vi "Encoded 2D gaussian.vi"(5 "Coefficients":dbl[](array[numeric]) format="%.5f", 6 "X":dbl format="%.3f", 7 "code":dbl format="%.2f", 8 "fit type":u16, 9 "Flag":enum16{"no deriv", "deriv"}(ring)) -> (0 "Derivatives":dbl[](array[numeric]) format="%.5f", 2 "Y":dbl format="%.3f")   [LabVIEW 2011]
doc: "Evaluates the fit function at a point given the specified coefficients (i.e., fit parameters). Code is the value used to convert a raster-encoded 2-D position (which is what is supplied to this function by its caller) into a true 2-D position (which is what the equations for the function need to use).\n\nIf the partial derivatives of the function are known, the user also furnishes the equations for the partial derivatives of this function with respect to each coefficient. The input control Flag should then be set to 1 (deriv) by all calling VIs.\n\nIf the partial derivatives of the function are not known, the input control Flag should be set to 0 (no deriv) by all calling VIs, and a numerical approximation to the partial derivatives will be computed."
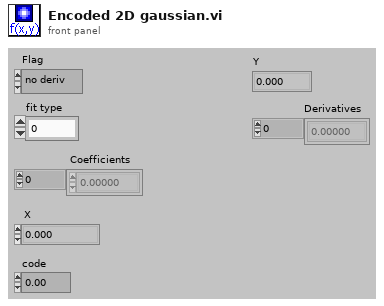
[diagram p1: front panel]
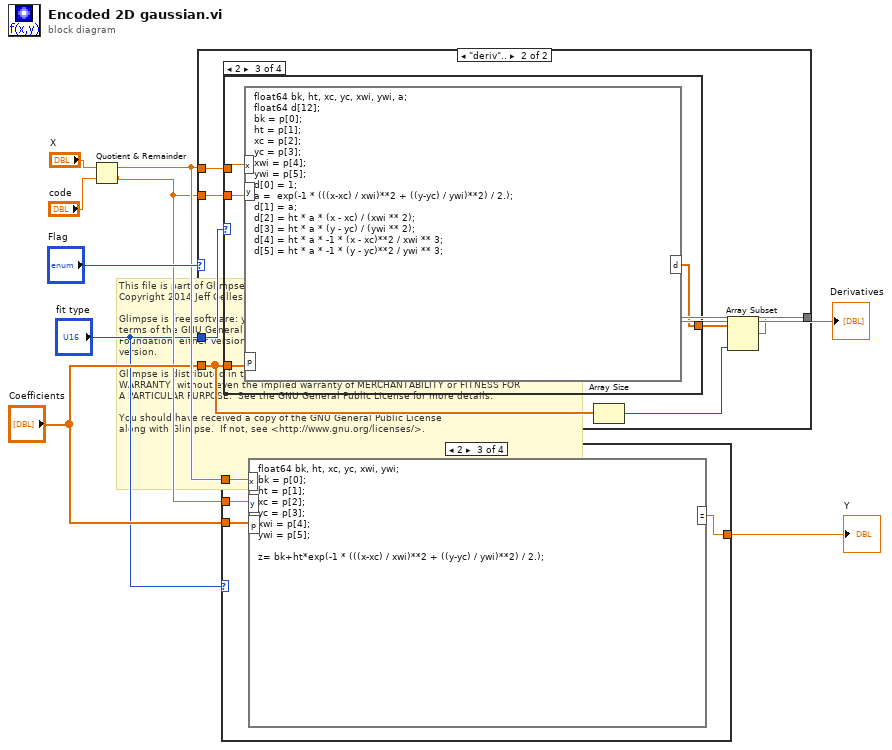
[diagram p0: block diagram]
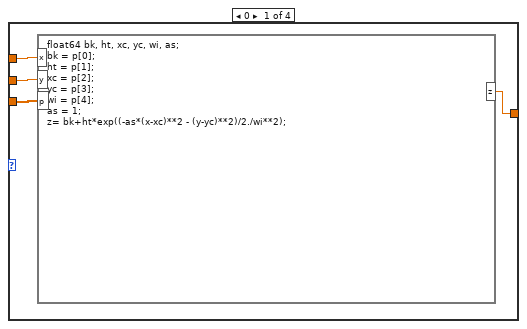
[diagram p2: hidden frame]
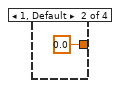
[diagram p3: hidden frame]
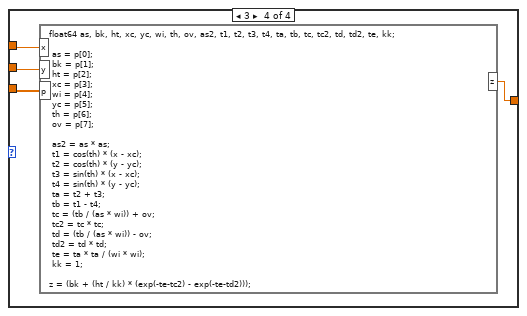
[diagram p4: hidden frame]
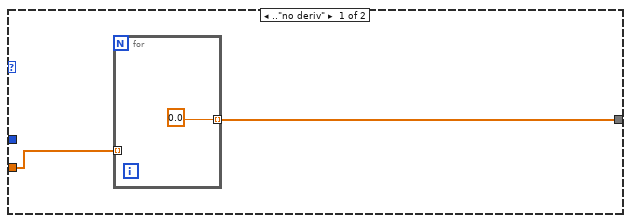
[diagram p5: hidden frame]
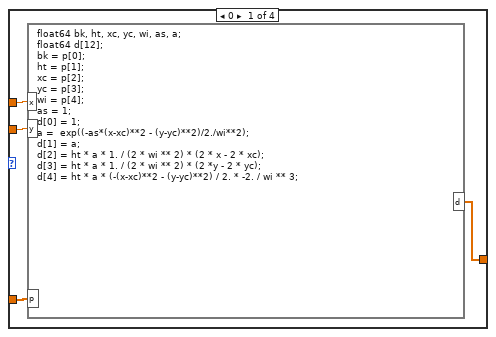
[diagram p6: hidden frame]
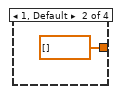
[diagram p7: hidden frame]
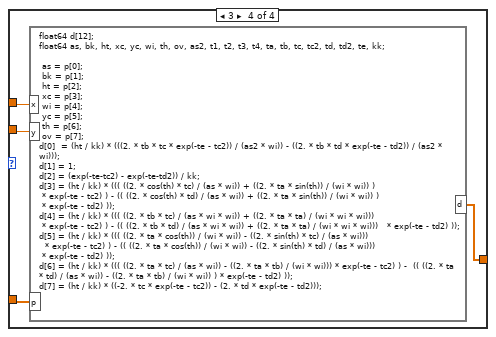
[diagram p8: hidden frame]
diagram:
  # "This file is part of Glimpse. \nCopyright 2014 Jeff Gelles, Brandeis University.    \n\nGlimpse is free software: you can redistribute it and/or modify it under the \nterms of the GNU General Public License as published by the Free Software \nFoundation, either version 3 of the License, or (at your option) any later \nversion.\n\nGlimpse is distributed in the hope that it will be useful, but WITHOUT ANY \nWARRANTY; without even the implied warranty of MERCHANTABILITY or FITNESS FOR \nA PARTICULAR PURPOSE.  See the GNU General Public License for more details.\n\nYou should have received a copy of the GNU General Public License\nalong with Glimpse.  If not, see <http://www.gnu.org/licenses/>."
  n1 = Quotient & Remainder(x="X", y="code") -> (x-y*floor(x/y)=w5:dbl, floor(x/y)=w2:dbl)
  n2 = case shown="\"deriv\".." "Flag" {
    tunnel: w5 -> [_ w19]
    tunnel: "Coefficients" -> [w11 w17]
    tunnel: [w10 w14] -> w3
    tunnel: w2 -> [_ w18]
    tunnel: "fit type" -> [_ w13]
    frame .."no deriv" {
      n3 = for {
        tunnel: w11 -> [_] mode=indexing
        tunnel: [0.0] -> w10 mode=indexing
      }
    }
    frame "deriv".. {
      n4 = case shown="2" w13 {
        tunnel: w19 -> [w23 _ w28 w32]
        tunnel: w18 -> [w22 _ w27 w31]
        tunnel: w17 -> [w21 _ w26 w30]
        tunnel: [w20 dbl[] [] w25 w29] -> w15
        frame 0 {
          n5 = formula code="float64 bk, ht, xc, yc, wi, as, a;\nfloat64 d[12];\nbk = p[0];\nht = p[1];\nxc = p[2];\nyc = p[3];\nwi = p[4];\nas = 1;\nd[0] = 1;\na =  exp((-as*(x-xc)**2 - (y-yc)**2)/2./wi**2);\nd[1] = a;\nd[2] = ht * a * 1. / (2 * wi ** 2) * (2 * x - 2 * xc);\nd[3] = ht * a * 1. / (2 * wi ** 2) * (2 *y - 2 * yc);\nd[4] = ht * a * (-(x-xc)**2 - (y-yc)**2) / 2. * -2. / wi ** 3;" ("Partial Derivatives of f(x) with respect to the coefficients p.")("x"=w23, "p"=w21, "y"=w22) -> ("d"=w20:dbl[])
        }
        frame 1, Default {
        }
        frame 2 {
          n6 = formula code="float64 bk, ht, xc, yc, xwi, ywi, a;\nfloat64 d[12];\nbk = p[0];\nht = p[1];\nxc = p[2];\nyc = p[3];\nxwi = p[4];\nywi = p[5];\nd[0] = 1;\na =  exp(-1 * (((x-xc) / xwi)**2 + ((y-yc) / ywi)**2) / 2.);\nd[1] = a;\nd[2] = ht * a * (x - xc) / (xwi ** 2);\nd[3] = ht * a * (y - yc) / (ywi ** 2);\nd[4] = ht * a * -1 * (x - xc)**2 / xwi ** 3;\nd[5] = ht * a * -1 * (y - yc)**2 / ywi ** 3;" ("Partial Derivatives of f(x) with respect to the coefficients p.")("x"=w28, "p"=w26, "y"=w27) -> ("d"=w25:dbl[])
        }
        frame 3 {
          n7 = formula code="float64 d[12];\nfloat64 as, bk, ht, xc, yc, wi, th, ov, as2, t1, t2, t3, t4, ta, tb, tc, tc2, td, td2, te, kk;\n\n\tas = p[0];\t\n\tbk = p[1];\t\n\tht = p[2];\t\n\txc = p[3];\t\n\twi = p[4];\t\n\tyc = p[5];\t\n\tth = p[6];\t\n\tov = p[7];\t\nd[0]  = (ht / kk) * (((2. * tb * tc * exp(-te - tc2)) / (as2 * wi)) - ((2. * tb * td * exp(-te - td2)) / (as2 * wi)));\nd[1] = 1;\nd[2] = (exp(-te-tc2) - exp(-te-td2)) / kk;\nd[3] = (ht / kk) * ((( ((2. * cos(th) * tc) / (as * wi)) + ((2. * ta * sin(th)) / (wi * wi)) )\n\t* exp(-te - tc2) ) - (( ((2. * cos(th) * td) / (as * wi)) + ((2. * ta * sin(th)) / (wi * wi)) )\n\t* exp(-te - td2) ));\nd[4] = (ht / kk) * ((( ((2. * tb * tc) / (as * wi * wi)) + ((2. * ta * ta) / (wi * wi * wi)))\n * exp(-te - tc2) ) - (( ((2. * tb * td) / (as * wi * wi)) + ((2. * ta * ta) / (wi * wi * wi)))   * exp(-te - td2) ));\nd[5] = (ht / kk) * ((( ((2. * ta * cos(th)) / (wi * wi)) - ((2. * sin(th) * tc) / (as * wi)))\n\t\t* exp(-te - tc2) ) - (( ((2. * ta * cos(th)) / (wi * wi)) - ((2. * sin(th) * td) / (as * wi)))\n\t* exp(-te - td2) ));\nd[6] = (ht / kk) * ((( ((2. * ta * tc) / (as * wi)) - ((2. * ta * tb) / (wi * wi))) * exp(-te - tc2) ) -  (( ((2. * ta * td) / (as * wi)) - ((2. * ta * tb) / (wi * wi)) ) * exp(-te - td2) ));\nd[7] = (ht / kk) * ((-2. * tc * exp(-te - tc2)) -\t(2. * td * exp(-te - td2)));" ("Partial Derivatives of f(x) with respect to the coefficients p.")("x"=w32, "p"=w30, "y"=w31) -> ("d"=w29:dbl[])
        }
      }
      n8 = Array Size(array=w17) -> (size(s)=w16:i32)
      n9 = Array Subset(array=w15, length=w16) -> (w14:dbl[])  [unwired: 1 in]
    }
  }
  "Derivatives" <- w3
  n10 = case shown="2" "fit type" {
    tunnel: [w36 0.0 ("z") w38 w42] -> w9
    tunnel: w5 -> [w35 _ w41 w45]
    tunnel: "Coefficients" -> [w34 _ w39 w43]
    tunnel: w2 -> [w33 _ w40 w44]
    frame 0 {
      n11 = formula code="float64 bk, ht, xc, yc, wi, as;\nbk = p[0];\nht = p[1];\nxc = p[2];\nyc = p[3];\nwi = p[4];\nas = 1;\nz= bk+ht*exp((-as*(x-xc)**2 - (y-yc)**2)/2./wi**2);" ("Function f(x)")("x"=w35, "y"=w33, "p"=w34) -> ("z"=w36:dbl)
    }
    frame 1, Default {
    }
    frame 2 {
      n12 = formula code="float64 bk, ht, xc, yc, xwi, ywi;\nbk = p[0];\nht = p[1];\nxc = p[2];\nyc = p[3];\nxwi = p[4];\nywi = p[5];\n\nz= bk+ht*exp(-1 * (((x-xc) / xwi)**2 + ((y-yc) / ywi)**2) / 2.);" ("Function f(x)")("x"=w41, "y"=w40, "p"=w39) -> ("z"=w38:dbl)
    }
    frame 3 {
      n13 = formula code="float64 as, bk, ht, xc, yc, wi, th, ov, as2, t1, t2, t3, t4, ta, tb, tc, tc2, td, td2, te, kk;\n\n\tas = p[0];\t\n\tbk = p[1];\t\n\tht = p[2];\t\n\txc = p[3];\t\n\twi = p[4];\t\n\tyc = p[5];\t\n\tth = p[6];\t\n\tov = p[7];\t\n\n\tas2 = as * as;\n\tt1 = cos(th) * (x - xc);\n\tt2 = cos(th) * (y - yc);\n\tt3 = sin(th) * (x - xc);\n\tt4 = sin(th) * (y - yc);\n\tta = t2 + t3;\n\ttb = t1 - t4;\n\ttc = (tb / (as * wi)) + ov;\n\ttc2 = tc * tc;\n\ttd = (tb / (as * wi)) - ov;\n\ttd2 = td * td;\n\tte = ta * ta / (wi * wi);\n\tkk = 1;\n\nz = (bk + (ht / kk) * (exp(-te-tc2) - exp(-te-td2)));" ("Function f(x)")("x"=w45, "y"=w44, "p"=w43) -> ("z"=w42:dbl)
    }
  }
  "Y" <- w9
